vi "Load2dArrayToSecList.vi"(8 "error in (no error)":errorcluster, 10 "Item Names":string[][](array[string]), 11 "GUI_Handler in":refnum<class "GUI_Handler.lvclass">) -> (0 "error out":errorcluster, 3 "GUI_Handler out":refnum<class "GUI_Handler.lvclass">)   [LabVIEW 2019, in "GUI_Handler.lvclass"]
uses:
  GUI_Handler.lvclass
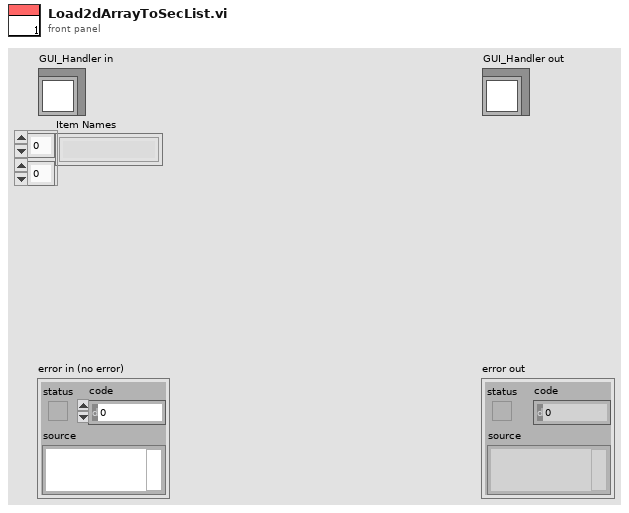
[diagram p1: front panel]
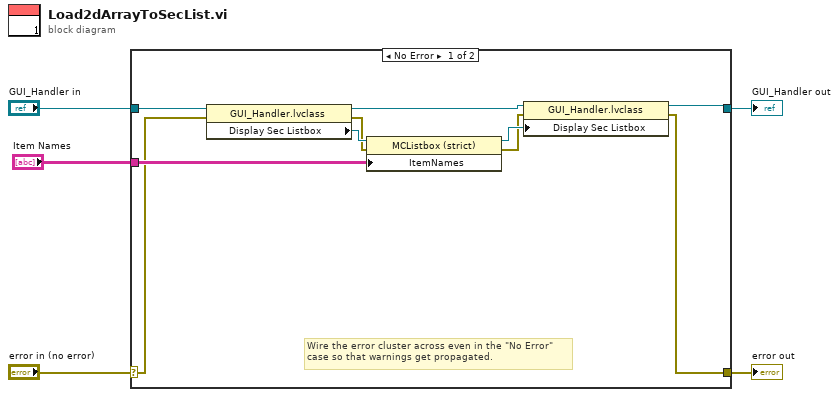
[diagram p0: block diagram]
diagram:
  n1 = case shown="No Error" "error in (no error)" {
    selector: "error in (no error)" -> [w10 w17]
    tunnel: [w6 w17] -> w4
    tunnel: [w7 w16] -> w2
    tunnel: "GUI_Handler in" -> [w15 w16]
    tunnel: "Item Names" -> [w13 _]
    frame No Error {
      # "Wire the error cluster across even in the \"No Error\"\ncase so that warnings get propagated."
      n2 = property class="GUI_Handler.lvclass"(reference=w15, error in=w10) -> (reference out=w12:refnum<class "GUI_Handler.lvclass">, error out=w9:errorcluster, "Display Sec Listbox"=w14:refnum<vi>)
      n3 = property class="MCListbox (strict)"(reference=w14, error in=w9, "ItemNames"=w13) -> (reference out=w11:refnum<vi>, error out=w8:errorcluster)
      n4 = property class="GUI_Handler.lvclass"(reference=w12, error in=w8, "Display Sec Listbox"=w11) -> (reference out=w7:refnum<class "GUI_Handler.lvclass">, error out=w6:errorcluster)
    }
    frame Error {
    }
  }
  "error out" <- w4
  "GUI_Handler out" <- w2
